vi "GPS Time to Timestamp.vi"(10 "Fractional Second":dbl, 11 "GPS Time (s)":i64) -> (1 "Not a Timestamp?":bool, 3 "Timestamp":timestamp)   [LabVIEW 2018]
uses:
  <vilib>/LabVIEW Open Source Project/Epoch Date & Time/epoch.GPS/Epoch.GPS.lvclass
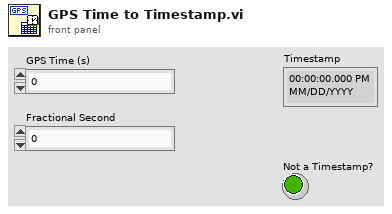
[diagram p1: front panel]
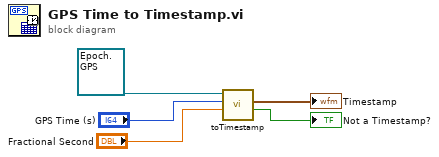
[diagram p0: block diagram]
diagram:
  n1 = call-dynamic "toTimestamp.vi"("Fractional Second"="Fractional Second", "GPS Time (s)"="GPS Time (s)", "Epoch (GPS)"=refnum<class "Epoch.GPS.lvclass"> refnum ("Epoch.GPS.lvclass")) -> ("Not a Timestamp?"=→"Not a Timestamp?":bool, "Timestamp"=→"Timestamp":timestamp)  [unwired: 6 in, 1 out]
